vi "EditOptions.vi"(8 "error in":errorcluster, 11 "LED editor node in":refnum<class "LED editor node.lvclass">) -> (0 "error out":errorcluster, 1 "edit options":T1, 2 "subnodes class":T2, 3 "LED editor node out":refnum<class "LED editor node.lvclass">)   [LabVIEW 2014, in "LED editor node.lvclass"]
doc: "This VI Contains the options for the Menu that will be displayed when doing right click on an item\nThe subnodes class configures which nodes can be added to this nodes\nAnd the edit options determine which options are available for the node.\n\nThis configuration is stored in this VI in case some dynamic configuration is required for the menu options or subnodes.\n\nAll VIs must overide this method"
uses:
  LED editor node.lvclass
  <vilib>/NI/Configuration Framework/Node/SubNodeCluster.ctl
  <vilib>/NI/Configuration Framework/Node/NodeMenuOptions.ctl
  <vilib>/NI/DCAF/Tag Editor Core/control module/editor node/control module editor.lvclass
  <vilib>/NI/Configuration Framework/Node/NISE_CEF_Node.lvclass
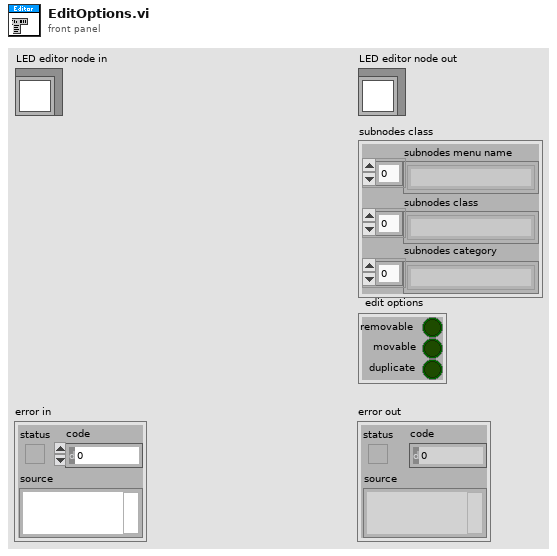
[diagram p1: front panel]
types:
  T1 = typedef "NISE_CEF_Node.lvclass/NodeMenuOptions.ctl" = cluster{"removable":bool, "movable":bool, "duplicate":bool}
  T2 = typedef "NISE_CEF_Node.lvclass/SubNodeCluster.ctl" = cluster{"subnodes menu name":string[], "subnodes class":string[], "subnodes category":string[]}
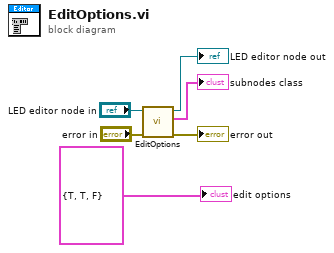
[diagram p0: block diagram]
diagram:
  n1 = call-parent "EditOptions.vi"("error in"="error in", "Module Editor Node in"="LED editor node in") -> ("error out"=→"error out":errorcluster, "subnodes class"=→"subnodes class":T2, "Module Editor Node out"=→"LED editor node out":refnum<class "LED editor node.lvclass">)  [unwired: 6 in, 1 out]
  "edit options" <- T1 {"removable"=TRUE, "movable"=TRUE, "duplicate"=FALSE} ("edit options")
